vi "SigInfo AcqSigRmk.vi"(8 "error in (no error)":errorcluster, 10 "signal in":waveform(sgl)) -> (0 "error out":errorcluster, 2 "signal out":waveform(sgl), 5 "sys_value_param":T1)   [LabVIEW 2018, in "SigInfo.lvclass"]
uses:
  SigInfo.lvclass
  RT/PublicSubVI/Ctl/_ctl_RT_ExpCondi.ctl
  SigInfo.lvclass/SigInfo.ctl
  <vilib>/Utility/error.llb/Error Cluster From Error Code.vi
  Overload/Experiment Condition/_PC_Pub_ExpCondiValue_Pressure.vi
  Overload/Experiment Condition/_PC_Pub_ExpCondiValue_Laser.vi
  Overload/Experiment Condition/_PC_Pub_ExpCondiValue_TMP.vi
  Overload/Experiment Condition/_PC_Pub_ExpCondiValue_SignalRemarks.vi
  <vilib>/ErrorRing/Error Ring.xnode
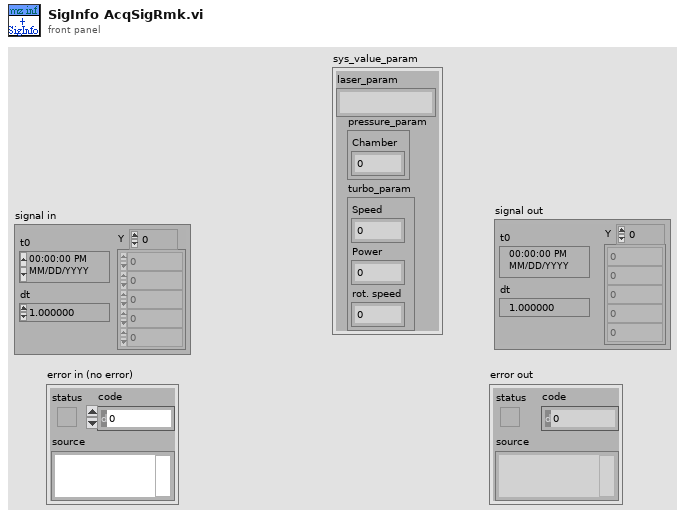
[diagram p1: front panel]
types:
  T1 = cluster{"laser_param":string, "pressure_param":cluster{"Chamber":dbl}, "turbo_param":cluster{"Speed":dbl, "Power":dbl, "rot. speed":dbl}}
  T2 = typedef "_ctl_RT_ExpCondi.ctl" = cluster{"Label":string, "Value":variant}[]
  T3 = cluster{"Speed":dbl, "Power":dbl, "rot. speed":dbl}
  T4 = cluster{"mzID":u64, "SignalInfo":cluster{"Label":string, "dt":dbl, "Length":u32, "RefVolt":dbl, "mzTable":cluster{"t":dbl[], "mz":dbl[], "beta":dbl[]}}[]}[]
  T5 = cluster{"InfoID":u64, "SignalInfo":cluster{"Label":string, "dt":dbl, "Length":u32, "RefVolt":dbl, "mzTable":cluster{"t":dbl[], "mz":dbl[], "beta":dbl[]}}[]}
  T6 = cluster{"Label":string, "dt":dbl, "Length":u32, "RefVolt":dbl, "mzTable":cluster{"t":dbl[], "mz":dbl[], "beta":dbl[]}}[]
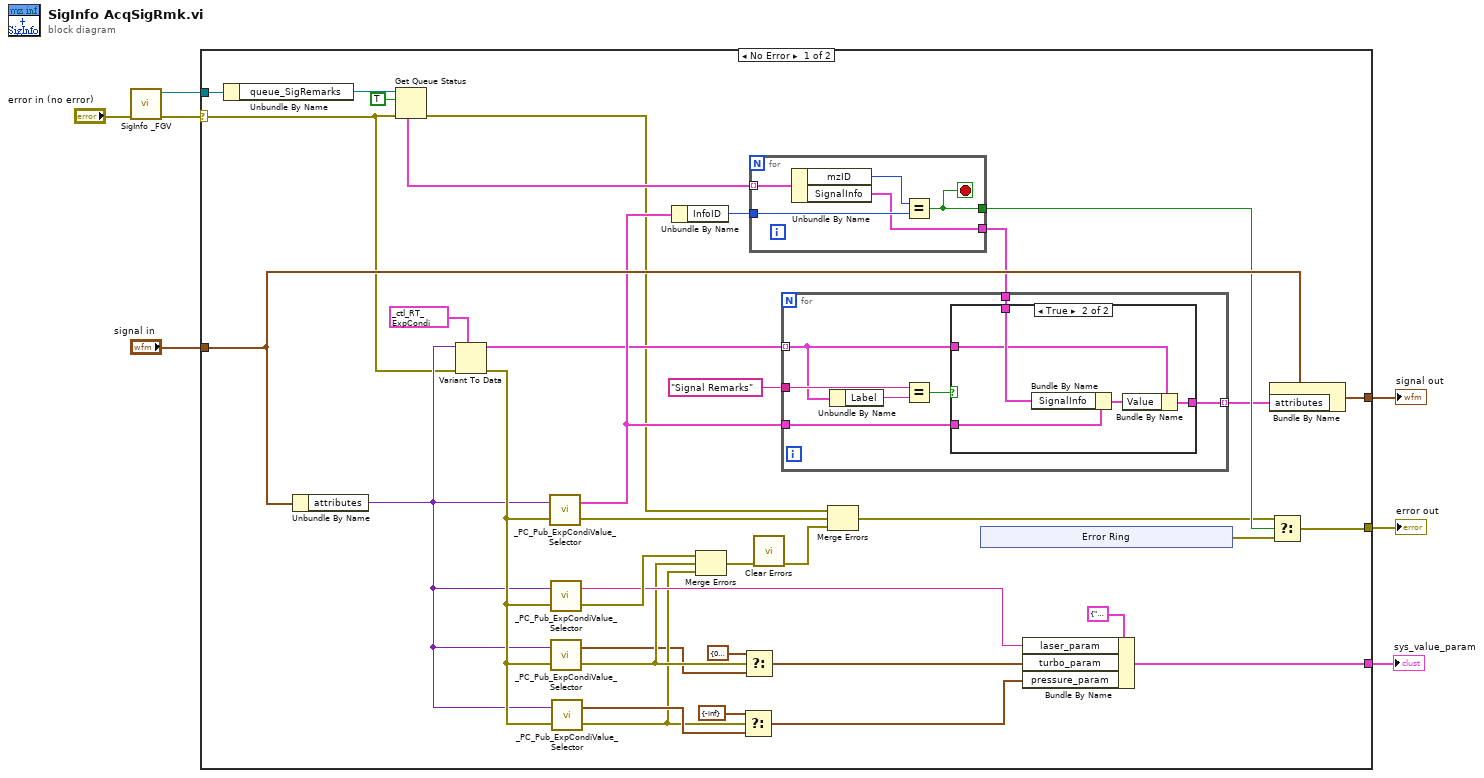
[diagram p0: block diagram]
diagram:
  n1 = call "SigInfo _FGV.vi"("error in (no error)"="error in (no error)") -> ("error out"=w4:errorcluster, "mzInfo out"=w6:refnum<class "SigInfo.lvclass">)  [unwired: 9 in]
  n2 = case shown="No Error" w4 {
    selector: w4 -> [w9 w66]
    tunnel: [w37 w66] -> w7
    tunnel: w6 -> [w42 _]
    tunnel: "signal in" -> [w43 _]
    tunnel: [w33 _] -> w2
    tunnel: [w25 _] -> w1
    frame No Error {
      n3 = Unbundle By Name(w42) -> ("queue_SigRemarks"=w41:refnum<queue>)
      n4 = Unbundle By Name(w43) -> ("attributes"=w10:variant)
      n5 = Get Queue Status(queue=w41, return elements? (F)=TRUE, error in (no error)=w9) -> (error out=w8:errorcluster, elements=w39:T4)  [unwired: 6 out]
      n6 = Variant To Data(error in=w9, type=T2 [{"Label"="Laser", "Value"=variant}, {"Label"="Pressure", "Value"=variant}, {"Label"="TMP", "Value"=variant}, {"Label"="Script", "Value"=variant}, {"Label"="Signal Remarks", "Value"=variant}, {"Label"="ExtAO", "Value"=variant}, {"Label"="ExtDO", "Value"=variant}, {"Label"="ExtDI", "Value"=variant}, {"Label"="D999", "Value"=variant}] ("ExpCondi"), Variant=w10) -> (data=w29:T2, error out=w28:errorcluster)
      n7 = call-poly "_PC_Pub_ExpCondiValue_Selector.vi"("error in (no error)"=w28, "expCondiVariant"=w10) -> ("error out"=w22:errorcluster, "SignalRemarks"=w32:T5)
      n8 = call-poly "_PC_Pub_ExpCondiValue_Selector.vi"("error in (no error)"=w28, "expCondiVariant"=w10) -> ("error out"=w30:errorcluster, "laserParam"=w26:string)
      n9 = call-poly "_PC_Pub_ExpCondiValue_Selector.vi"("error in (no error)"=w28, "expCondiVariant"=w10) -> ("error out"=w20:errorcluster, "TMP"=w14:T3)
      n10 = call-poly "_PC_Pub_ExpCondiValue_Selector.vi"("error in (no error)"=w28, "expCondiVariant"=w10) -> ("error out"=w17:errorcluster, "Pressure"=w18:cluster{"Chamber":dbl})
      n11 = Unbundle By Name(w32) -> ("InfoID"=w36:u64)
      n12 = Merge Errors(w30, w20, w17) -> (w24:errorcluster)
      n13 = Select(t=cluster{"Chamber":dbl} {"Chamber"=-inf}, s=w17, f=w18) -> (s? t:f=w16:cluster{"Chamber":dbl})
      n14 = Select(t=T3 {"Speed"=0.0, "Power"=0.0, "rot. speed"=0.0}, s=w20, f=w14) -> (s? t:f=w19:T3)
      n15 = for {
        tunnel: w39 -> [w63] mode=indexing
        tunnel: w36 -> [w64]
        tunnel: [w62] -> w38
        tunnel: [w61] -> w35
        stop <- w62 stop-if-true
        n16 = Unbundle By Name(w63) -> ("mzID"=w65:u64, "SignalInfo"=w61:T6)
        n17 = Equal?(x=w65, y=w64) -> (x = y?=w62:bool)
      }
      n18 = call <vilib>:"Clear Errors.vi"("error in (no error)"=w24) -> ("error out"=w23:errorcluster)  [unwired: 5 in, 1 out]
      n19 = for {
        tunnel: w29 -> [w51] mode=indexing
        tunnel: "Signal Remarks" -> [w53]
        tunnel: w32 -> [w49]
        tunnel: w35 -> [w50]
        tunnel: [w48] -> w34 mode=indexing
        n20 = Unbundle By Name(w51) -> ("Label"=w54:string)
        n21 = Equal?(x=w53, y=w54) -> (x = y?=w52:bool)
        n22 = case shown="True" w52 {
          tunnel: w51 -> [w55 w58]
          tunnel: w50 -> [_ w60]
          tunnel: w49 -> [_ w56]
          tunnel: [w55 w57] -> w48
          frame False {
          }
          frame True {
            n23 = Bundle By Name(cluster=w56, "SignalInfo"=w60) -> (w59:T5)
            n24 = Bundle By Name(cluster=w58, "Value"=w59) -> (w57:cluster{"Label":string, "Value":variant})
          }
        }
      }
      n25 = Merge Errors(w8, w22, w23) -> (w21:errorcluster)
      n26 = xnode "Error Ring"() -> ("error out"=w31:errorcluster)
      n27 = Bundle By Name(cluster=T1 {"laser_param"="", "pressure_param"={"Chamber"=0.0}, "turbo_param"={"Speed"=0.0, "Power"=0.0, "rot. speed"=0.0}}, "laser_param"=w26, "turbo_param"=w19, "pressure_param"=w16) -> (w25:T1)
      n28 = Bundle By Name(cluster=w43, "attributes"=w34) -> (w33:waveform(sgl))
      n29 = Select(t=w21, s=w38, f=w31) -> (s? t:f=w37:errorcluster)
    }
    frame Error {
    }
  }
  "error out" <- w7
  "signal out" <- w2
  "sys_value_param" <- w1
